vi "Text-Starts With.vi"(4 "Starts with":string, 5 "String":string) -> (1 "result":bool)   [LabVIEW 2020]
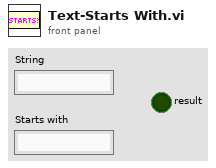
[diagram p1: front panel]
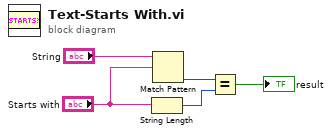
[diagram p0: block diagram]
diagram:
  n1 = String Length(string="Starts with") -> (length=w2:i32)
  n2 = Match Pattern(string="String", regular expression="Starts with") -> (offset past match=w3:i32)  [unwired: 1 in, 3 out]
  n3 = Equal?(x=w3, y=w2) -> (x = y?=→"result":bool)
